vi "GW_2FC_ctl.vi"(8 "error in":errorcluster caption="错误输入（无错误）", 9 "Input2":T2, 11 "Input1":T3) -> (0 "error out":errorcluster caption="错误输出", 1 "GW2FC":T1 {"PEPS电源模式" items=["OFF", "ACC", "ON", "Reserved", "START", "Reserved", "Reserved", "Reserved"]; "PEPS电源模式有效指示" items=["Not available", "Invalid", "Valid", "Reserved"]}, 3 "CmdStr":string)   [LabVIEW 2013]
uses:
  Input1.ctl
  Input2.ctl
  GW_PEPS_2FC.ctl
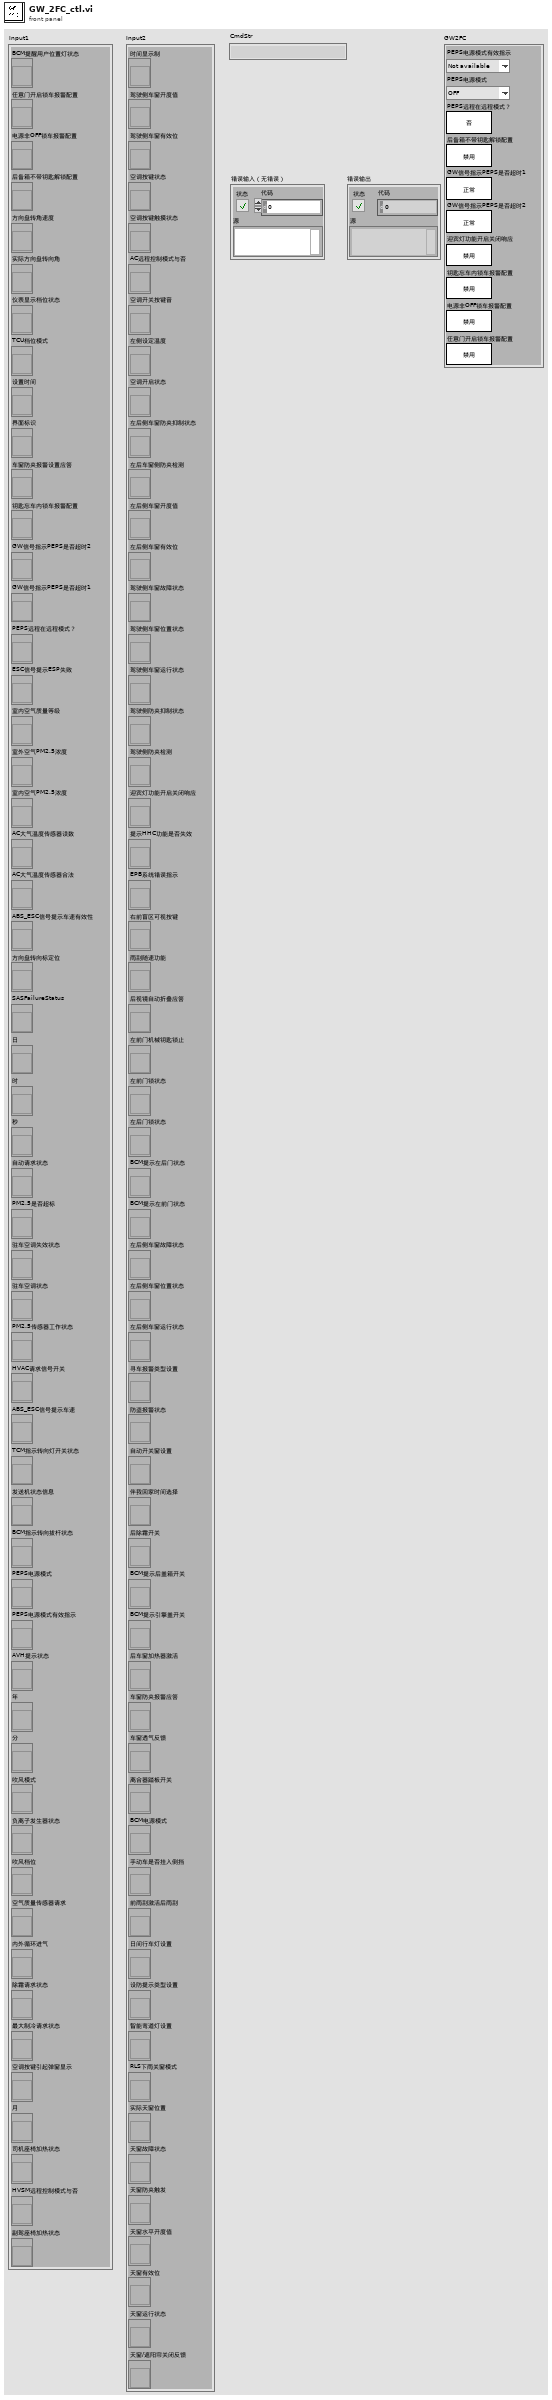
[diagram p1: front panel]
types:
  T1 = typedef "GW_PEPS_2FC.ctl" = cluster{"PEPS电源模式有效指示":u16, "PEPS电源模式":u16, "PEPS远程在远程模式？":bool, "后备箱不带钥匙解锁配置":bool, "GW信号指示PEPS是否超时1":bool, "GW信号指示PEPS是否超时2":bool, "迎宾灯功能开启关闭响应":bool, "钥匙忘车内锁车报警配置":bool, "电源非OFF锁车报警配置":bool, "任意门开启锁车报警配置":bool}
  T2 = typedef "Input2.ctl" = cluster{"时间显示制":refnum<vi>, "驾驶侧车窗开度值":refnum<vi>, "驾驶侧车窗有效位":refnum<vi>, "空调按键状态":refnum<vi>, "空调按键触摸状态":refnum<vi>, "AC远程控制模式与否":refnum<vi>, "空调开关按键音":refnum<vi>, "左侧设定温度":refnum<vi>, "空调开启状态":refnum<vi>, "左后侧车窗防夹抑制状态":refnum<vi>, "左后车窗侧防夹检测":refnum<vi>, "左后侧车窗开度值":refnum<vi>, "左后侧车窗有效位":refnum<vi>, "驾驶侧车窗故障状态":refnum<vi>, "驾驶侧车窗位置状态":refnum<vi>, "驾驶侧车窗运行状态":refnum<vi>, "驾驶侧防夹抑制状态":refnum<vi>, "驾驶侧防夹检测":refnum<vi>, "迎宾灯功能开启关闭响应":refnum<vi>, "提示HHC功能是否失效":refnum<vi>, "EPB系统错误指示":refnum<vi>, "右前盲区可视按键":refnum<vi>, "雨刮随速功能":refnum<vi>, "后视镜自动折叠应答":refnum<vi>, "左前门机械钥匙锁止":refnum<vi>, "左前门锁状态":refnum<vi>, "左后门锁状态":refnum<vi>, "BCM提示左后门状态":refnum<vi>, "BCM提示左前门状态":refnum<vi>, "左后侧车窗故障状态":refnum<vi>, "左后侧车窗位置状态":refnum<vi>, "左后侧车窗运行状态":refnum<vi>, "寻车报警类型设置":refnum<vi>, "防盗报警状态":refnum<vi>, "自动开关窗设置":refnum<vi>, "伴我回家时间选择":refnum<vi>, "后除霜开关":refnum<vi>, "BCM提示后盖箱开关":refnum<vi>, "BCM提示引擎盖开关":refnum<vi>, "后车窗加热器激活":refnum<vi>, "车窗防夹报警应答":refnum<vi>, "车窗透气反馈":refnum<vi>, "离合器踏板开关":refnum<vi>, "BCM电源模式":refnum<vi>, "手动车是否挂入倒挡":refnum<vi>, "前雨刮激活后雨刮":refnum<vi>, "日间行车灯设置":refnum<vi>, "设防提示类型设置":refnum<vi>, "智能弯道灯设置":refnum<vi>, "RLS下雨关窗模式":refnum<vi>, "实际天窗位置":refnum<vi>, "天窗故障状态":refnum<vi>, "天窗防夹触发":refnum<vi>, "天窗水平开度值":refnum<vi>, "天窗有效位":refnum<vi>, "天窗运行状态":refnum<vi>, "天窗/遮阳帘关闭反馈":refnum<vi>}
  T3 = typedef "Input1.ctl" = cluster{"BCM提醒用户位置灯状态":refnum<vi>, "任意门开启锁车报警配置":refnum<vi>, "电源非OFF锁车报警配置":refnum<vi>, "后备箱不带钥匙解锁配置":refnum<vi>, "方向盘转角速度":refnum<vi>, "实际方向盘转向角":refnum<vi>, "仪表显示档位状态":refnum<vi>, "TCU档位模式":refnum<vi>, "设置时间":refnum<vi>, "界面标识":refnum<vi>, "车窗防夹报警设置应答":refnum<vi>, "钥匙忘车内锁车报警配置":refnum<vi>, "GW信号指示PEPS是否超时2":refnum<vi>, "GW信号指示PEPS是否超时1":refnum<vi>, "PEPS远程在远程模式？":refnum<vi>, "ESC信号提示ESP失败":refnum<vi>, "室内空气质量等级":refnum<vi>, "室外空气PM2.5浓度":refnum<vi>, "室内空气PM2.5浓度":refnum<vi>, "AC大气温度传感器读数":refnum<vi>, "AC大气温度传感器合法":refnum<vi>, "ABS_ESC信号提示车速有效性":refnum<vi>, "方向盘转向标定位":refnum<vi>, "SASFailureStatus":refnum<vi>, "日":refnum<vi>, "时":refnum<vi>, "秒":refnum<vi>, "自动请求状态":refnum<vi>, "PM2.5是否超标":refnum<vi>, "驻车空调失效状态":refnum<vi>, "驻车空调状态":refnum<vi>, "PM2.5传感器工作状态":refnum<vi>, "HVAC请求信号开关":refnum<vi>, "ABS_ESC信号提示车速":refnum<vi>, "TCM指示转向灯开关状态":refnum<vi>, "发送机状态信息":refnum<vi>, "BCM指示转向拔杆状态":refnum<vi>, "PEPS电源模式":refnum<vi>, "PEPS电源模式有效指示":refnum<vi>, "AVH提示状态":refnum<vi>, "年":refnum<vi>, "分":refnum<vi>, "吹风模式":refnum<vi>, "负离子发生器状态":refnum<vi>, "吹风档位":refnum<vi>, "空气质量传感器请求":refnum<vi>, "内外循环进气":refnum<vi>, "除霜请求状态":refnum<vi>, "最大制冷请求状态":refnum<vi>, "空调按键引起弹窗显示":refnum<vi>, "月":refnum<vi>, "司机座椅加热状态":refnum<vi>, "HVSM远程控制模式与否":refnum<vi>, "副驾座椅加热状态":refnum<vi>}
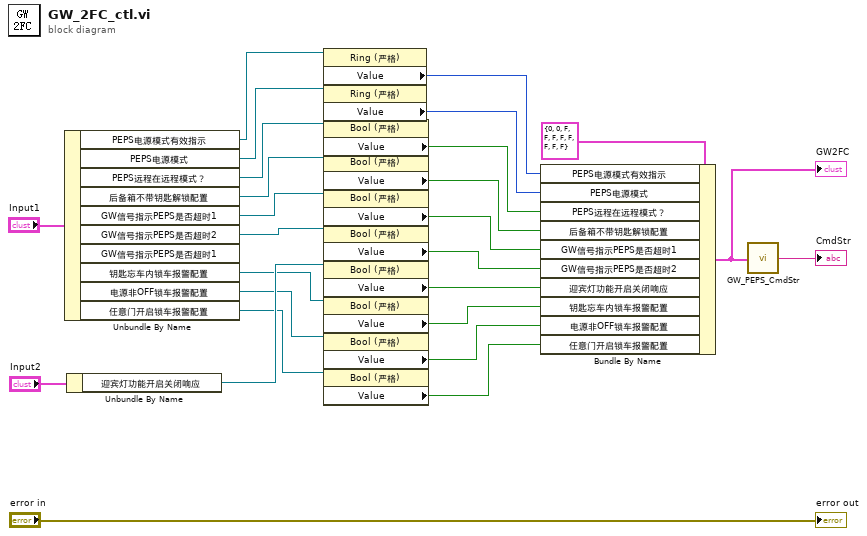
[diagram p0: block diagram]
diagram:
  n1 = Unbundle By Name("Input1") -> ("PEPS电源模式有效指示"=w23:refnum<vi>, "PEPS电源模式"=w21:refnum<vi>, "PEPS远程在远程模式？"=w19:refnum<vi>, "后备箱不带钥匙解锁配置"=w17:refnum<vi>, "GW信号指示PEPS是否超时1"=w15:refnum<vi>, "GW信号指示PEPS是否超时2"=w13:refnum<vi>, "钥匙忘车内锁车报警配置"=w9:refnum<vi>, "电源非OFF锁车报警配置"=w7:refnum<vi>, "任意门开启锁车报警配置"=w6:refnum<vi>)  [unwired: 1 out]
  n2 = Unbundle By Name("Input2") -> ("迎宾灯功能开启关闭响应"=w11:refnum<vi>)
  n3 = property class="Ring (严格)"(reference=w23) -> ("Value"=w22:u16)  [unwired: 1 in, 2 out]
  n4 = property class="Ring (严格)"(reference=w21) -> ("Value"=w20:u16)  [unwired: 1 in, 2 out]
  n5 = property class="Bool (严格)"(reference=w19) -> ("Value"=w18:bool)  [unwired: 1 in, 2 out]
  n6 = property class="Bool (严格)"(reference=w17) -> ("Value"=w16:bool)  [unwired: 1 in, 2 out]
  n7 = property class="Bool (严格)"(reference=w15) -> ("Value"=w14:bool)  [unwired: 1 in, 2 out]
  n8 = property class="Bool (严格)"(reference=w13) -> ("Value"=w12:bool)  [unwired: 1 in, 2 out]
  n9 = property class="Bool (严格)"(reference=w11) -> ("Value"=w10:bool)  [unwired: 1 in, 2 out]
  n10 = property class="Bool (严格)"(reference=w9) -> ("Value"=w8:bool)  [unwired: 1 in, 2 out]
  n11 = property class="Bool (严格)"(reference=w7) -> ("Value"=w5:bool)  [unwired: 1 in, 2 out]
  n12 = property class="Bool (严格)"(reference=w6) -> ("Value"=w4:bool)  [unwired: 1 in, 2 out]
  n13 = Bundle By Name(cluster=T1 {"PEPS电源模式有效指示"=0, "PEPS电源模式"=0, "PEPS远程在远程模式？"=FALSE, "后备箱不带钥匙解锁配置"=FALSE, "GW信号指示PEPS是否超时1"=FALSE, "GW信号指示PEPS是否超时2"=FALSE, "迎宾灯功能开启关闭响应"=FALSE, "钥匙忘车内锁车报警配置"=FALSE, "电源非OFF锁车报警配置"=FALSE, "任意门开启锁车报警配置"=FALSE} ("GW_PEPS信息"), "PEPS电源模式有效指示"=w22, "PEPS电源模式"=w20, "PEPS远程在远程模式？"=w18, "后备箱不带钥匙解锁配置"=w16, "GW信号指示PEPS是否超时1"=w14, "GW信号指示PEPS是否超时2"=w12, "迎宾灯功能开启关闭响应"=w10, "钥匙忘车内锁车报警配置"=w8, "电源非OFF锁车报警配置"=w5, "任意门开启锁车报警配置"=w4) -> (w2:T1)
  "GW2FC" <- w2
  n14 = call "GW_PEPS_CmdStr.vi"("GW_PEPS信息"=w2) -> ("CmdStr"=→"CmdStr":string)
  "error out" <- "error in"
